vi "IniToken Load From LabVIEW.ini.vi"(8 "error in (no error)":errorcluster, 11 "IniTokenCluster":T1) -> (0 "error out":errorcluster, 3 "Cluster":T2)   [LabVIEW 2017]
uses:
  <resource>/dialog/lvconfig.llb/LV Config Read String.vi
  Def-IniTokenCluster.ctl
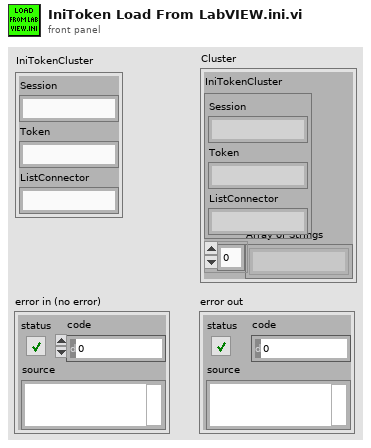
[diagram p1: front panel]
types:
  T1 = typedef "Def-IniTokenCluster.ctl" = cluster{"Session":string, "Token":string, "ListConnector":string}
  T2 = cluster{"IniTokenCluster":T1, "Array of Strings":string[]}
  T3 = cluster{"IniTokenCluster":T1, "string array":string[]}
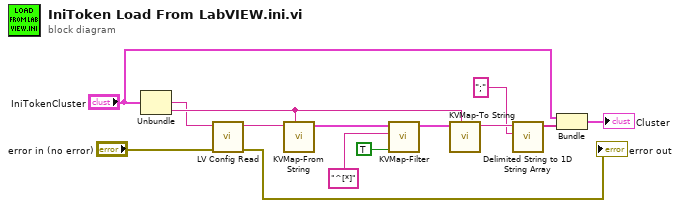
[diagram p0: block diagram]
diagram:
  n1 = Unbundle("IniTokenCluster") -> ("Token"=w8:string, "ListConnector"=w9:string)  [unwired: 1 out]
  n2 = call-poly <resource>:"LV Config Read.vi"("error in"="error in (no error)", "key"=w8) -> ("error out"=→"error out":errorcluster, "value"=w3:string)  [unwired: 3 in, 1 out]
  n3 = call "KVMap-From String.vi"("delimiter (Tab)"=w9, "value"=w3) -> ("Cluster"=w4:cluster{string[], string[]})  [unwired: 9 in]
  n4 = call "KVMap-Filter.vi"("T->First/F->Second(F)"=TRUE, "filter"="^[*]", "Cluster in"=w4) -> ("Cluster out"=w5:cluster{string[], string[]})  [unwired: 8 in]
  n5 = call "KVMap-To String.vi"("string"=w9, "Cluster"=w5) -> ("value"=w2:string)  [unwired: 9 in]
  n6 = call "Delimited String to 1D String Array.vi"("delimiter"=";" ("delimiter (Tab)"), "delimited string"=w2) -> ("string array"=w11:string[])  [unwired: 9 in]
  n7 = Bundle("IniTokenCluster"="IniTokenCluster", "string array"=w11) -> (→"Cluster":T3)  [unwired: 1 in]
